vi "Check Refnum Type.vi"(8 "error in (no error)":errorcluster, 11 "FK Ring in":refnum<class "FK Ring.lvclass">) -> (0 "error out":errorcluster, 3 "FK Ring out":refnum<class "FK Ring.lvclass">)   [LabVIEW 2020, in "Basic Fields.lvlib" / "FK Ring.lvclass"]
uses:
  FK Ring.lvclass
  Basic Fields/Basic Field Class/Ctrl Refnum Column.lvclass
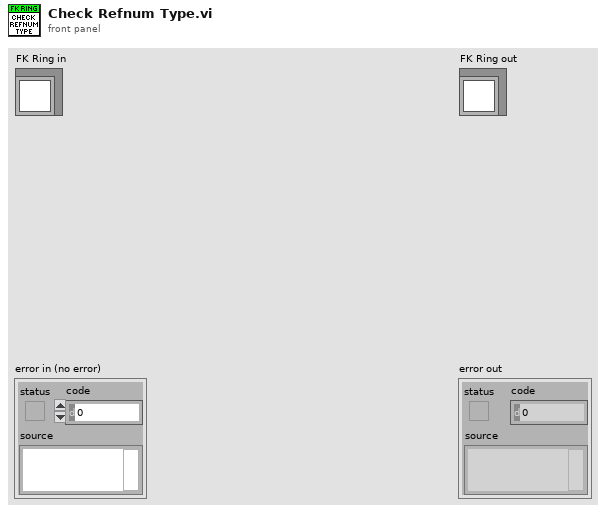
[diagram p1: front panel]
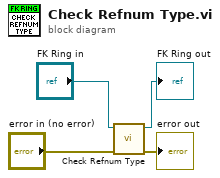
[diagram p0: block diagram]
diagram:
  n1 = call-parent "Check Refnum Type.vi"("error in (no error)"="error in (no error)", "Ctrl Refnum Column in"="FK Ring in") -> ("error out"=→"error out":errorcluster, "Ctrl Refnum Column out"=→"FK Ring out":refnum<class "FK Ring.lvclass">)  [unwired: 8 in]
